vi "Drive Shifter.vi"(8 "Button Index Low":i32=5, 9 "Button Index High":i32=4, 11 "Buttons":bool[](array[boolean])) -> (3 "High/Low":bool)   [LabVIEW 2014]
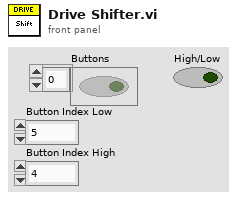
[diagram p1: front panel]
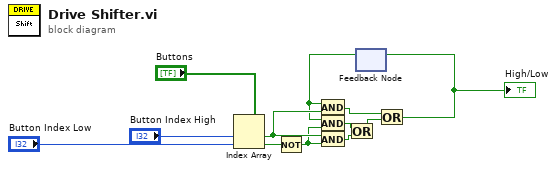
[diagram p0: block diagram]
diagram:
  n1 = Index Array(array="Buttons", index #1="Button Index High", index #2="Button Index Low") -> (element #1=w6:bool, element #2=w3:bool)
  n2 = Not(x=w3) -> (.not. x?=w4:bool)
  n3 = And(x=w6, y=w4) -> (x .and. y?=w8:bool)
  n4 = feedback #1() -> (w5:bool)  [unwired: 1 in]
  n5 = And(x=w5, y=w6) -> (x .and. y?=w11:bool)
  n6 = And(x=w5, y=w4) -> (x .and. y?=w7:bool)
  n7 = Or(x=w7, y=w8) -> (x .or. y?=w9:bool)
  n8 = Or(x=w11, y=w9) -> (x .or. y?=w10:bool)
  "High/Low" <- w10
  n9 = feedback-in #1(w10) -> ()
